vi "Refresh Targets_Do.vi"(8 "Error In":errorcluster, 9 "Tracking Progress bar":refnum<vi>, 10 "Allow UI?(T)":bool=TRUE, 11 "Dependency Source Plugins":refnum<class "Dependency Source.lvclass">[](array[class])) -> (0 "Error Out":errorcluster, 1 "All Success?":bool, 2 "Success? Array":bool[](array[boolean]))   [LabVIEW 2019, in "Project.Dependencies Finder.lvlib"]
doc: "Refresh target lists for the given Dependency Source Plugins.\nProvider a Tracker to have a live view of the progress.\n\n2020-12-07: Henrik Dueholm Hansen"
uses:
  Project.Dependencies Finder.lvlib
  Dependency Source/Dependency Source.lvclass
  Dependency Source/Dependency Source.lvclass/Dependency Source.ctl
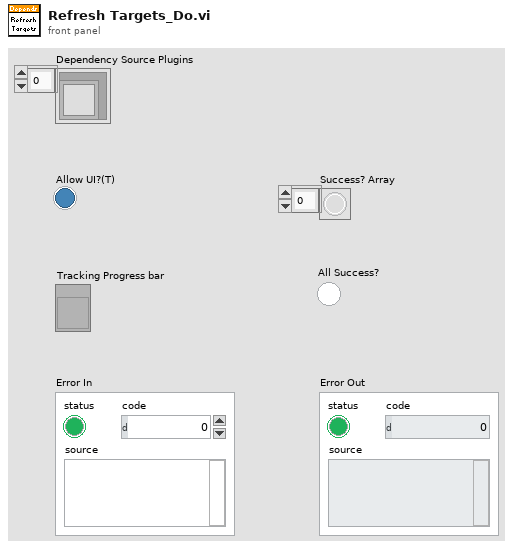
[diagram p1: front panel]
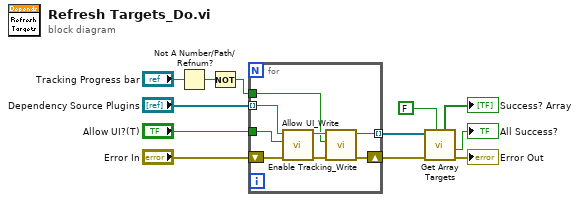
[diagram p0: block diagram]
diagram:
  n1 = Not A Number/Path/Refnum?(number/path/refnum="Tracking Progress bar") -> (NaN/Path/Refnum?=w2:bool)
  n2 = Not(x=w2) -> (.not. x?=w1:bool)
  n3 = for {
    tunnel: "Dependency Source Plugins" -> [w20] mode=indexing
    tunnel: [w14] -> w7 mode=indexing
    tunnel: "Allow UI?(T)" -> [w18]
    shift-right: [w16] -> w4
    shift-left: "Error In" -> [w19]
    tunnel: w1 -> [w13]
    n4 = call "Allow UI_Write.vi"("error in (no error)"=w19, "Allow UI?"=w18, "Dependency Source in"=w20) -> ("error out"=w17:errorcluster, "Dependency Source out"=w15:refnum<class "Dependency Source.lvclass">)  [unwired: 7 in]
    n5 = call "Enable Tracking_Write.vi"("error in (no error)"=w17, "Enable Tracking?"=w13, "Dependency Source in"=w15) -> ("error out"=w16:errorcluster, "Dependency Source out"=w14:refnum<class "Dependency Source.lvclass">)  [unwired: 7 in]
  }
  n6 = call "Get Array Targets.vi"("Load Stored Targets?(T)"=FALSE, "error in (no error)"=w4, "Dependency Sources"=w7) -> ("error out"=→"Error Out":errorcluster, "All Success?"=→"All Success?":bool, "Success? Array"=→"Success? Array":bool[])  [unwired: 3 in, 3 out]
